vi "chiller.vi"(11 "VISA Refnum in":refnum<visa-resource-name>) -> (3 "chiller actual temperature":string)   [LabVIEW 2019]
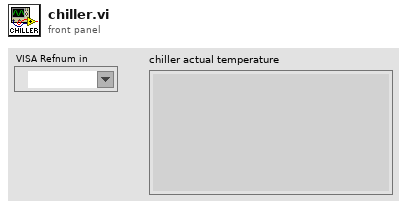
[diagram p1: front panel]
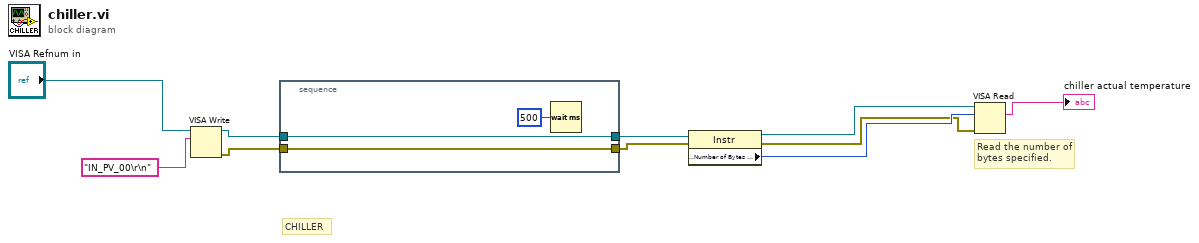
[diagram p0: block diagram]
diagram:
  # "CHILLER"
  # "Read the number of bytes specified."
  n1 = VISA Write(VISA resource name="VISA Refnum in", write buffer="IN_PV_00\r\n") -> (VISA resource name out=w2:refnum<visa-resource-name>, error out=w1:errorcluster)  [unwired: 1 in, 1 out]
  n2 = stacked-sequence {
    tunnel: w1 -> [w13]
    tunnel: [w13] -> w9
    tunnel: w2 -> [w12]
    tunnel: [w12] -> w8
    frame #0 {
      n3 = Wait (ms)(milliseconds to wait=u32 500) -> ()  [unwired: 1 out]
    }
  }
  n4 = property class="Instr"(reference=w8, error in=w9) -> (reference out=w3:refnum<visa-resource-name>, error out=w4:errorcluster, "Serial Settings:Number of Bytes at Serial Port"=w5:u32)
  n5 = VISA Read(VISA resource name=w3, byte count=w5, error in (no error)=w4) -> (read buffer=→"chiller actual temperature":string)  [unwired: 3 out]
